vi "PSK_Mod_Receive_queue_simplified.vi"() -> ()   [LabVIEW 2014]
uses:
  <vilib>/addons/Modulation/Digital/General/MT Generate Bits (Galois, PN Order).vi
  <vilib>/Analysis/2dsp.llb/1D Auto Correlation (DBL).vi
  <vilib>/addons/Modulation/Digital/Support/Common/Validators/mod_Generate Bits Validate.vi
  <vilib>/addons/Modulation/Analog/support/mod_Set Error Source.vi
  <vilib>/addons/Modulation/Digital/General/MT Generate PSK System Parameters(M).vi
  <vilib>/addons/Modulation/Digital/Support/Common/Validators/mod_Generate Filter Coefficients Validate.vi
  <vilib>/addons/Modulation/Digital/General/subVIs/mod_Generate Filter Coefficients.vi
  <vilib>/addons/Modulation/Digital/General/subVIs/mod_Generate Bits PN Sequence.vi
  <vilib>/addons/Modulation/Digital/General/MT Generate PSK Synchronization Parameters (bit array).vi
  <instrlib>/niUSRP/niUSRP Fetch Rx Data (CDB Cluster).vi
  <vilib>/addons/Modulation/Digital/General/MT Align to Ideal Symbols (Generic).vi
  <vilib>/addons/Modulation/Digital/General/MT Map PSK Symbols to Bits.vi
  <vilib>/Analysis/2dsp.llb/1D Cross Correlation (DBL).vi
  <vilib>/Utility/file.llb/Write To Spreadsheet File (I64).vi
  <vilib>/addons/Modulation/niDMT.lvlib
  <vilib>/Analysis/NI_AALPro.lvlib
panel:
  in  "stop 2":bool
  out "output bit stream":i8[](array[numeric])
  out "max index(es)":i32
  out "Bits received":i32
  out "Max Rxx Sync Sequence":dbl
  out "Numeric":i32
  in  "stop":bool
  out "USRP loop time":dbl
  in  "Header bits":i32=16
  out "Aquisition time":dbl
  in  "Message bits":i32=128
  in  "Sync bits":i32=30
  out "sync correct?":bool
  out "error out":errorcluster={"status"=FALSE, "code"=1074118647, "source"="niUSRP Fetch Rx Data (CDB Cluster).vi<ERR>Overflow: an internal receive buffer has filled before the data could be returned.  Consider reducing the IQ rate, increasing the Fetch rate, or increasing the number of samples per Fetch."}
  in  "USRP IP Address":refnum<k15>="192.168.10.1"
  out "Actual Rx Parameters":T1={"Rx IQ Sampling\nRate [s/sec]"=200000.0, "Rx\nFrequency [Hz]"=915000000.0, "Rx Gain [dB]"=20.0, "Rx Antenna"="RX1"} {"Rx Gain [dB]" format="%#.6p"; "Rx\nFrequency [Hz]" format="%#.6p"; "Rx IQ Sampling\nRate [s/sec]" format="%#.6p"}
  in  "Rx Parameters":T1={"Rx IQ Sampling\nRate [s/sec]"=400000.0, "Rx\nFrequency [Hz]"=5795000000.0, "Rx Gain [dB]"=0.0, "Rx Antenna"="RX1"} {"Rx Gain [dB]" format="%#.6p"; "Rx\nFrequency [Hz]" format="%#.6p"; "Rx IQ Sampling\nRate [s/sec]" format="%#.6p"}
  in  "Packets per burst":i32=20
  in  "filter parameters":T2={"Alpha"=0.5, "Filter Length"=6, "TX Filter"=enum."Root Raised Cos"} {"Alpha" format="%.2f"}
  in  "QPSK System Parameters":T3={"Samples per Symbol"=8, "symbol map"=[], "Differential PSK"=enum."disable", "PSK type"=0} {"PSK type" items=["normal", "shifted", "offset"]; "symbol map" format="%.3f"}
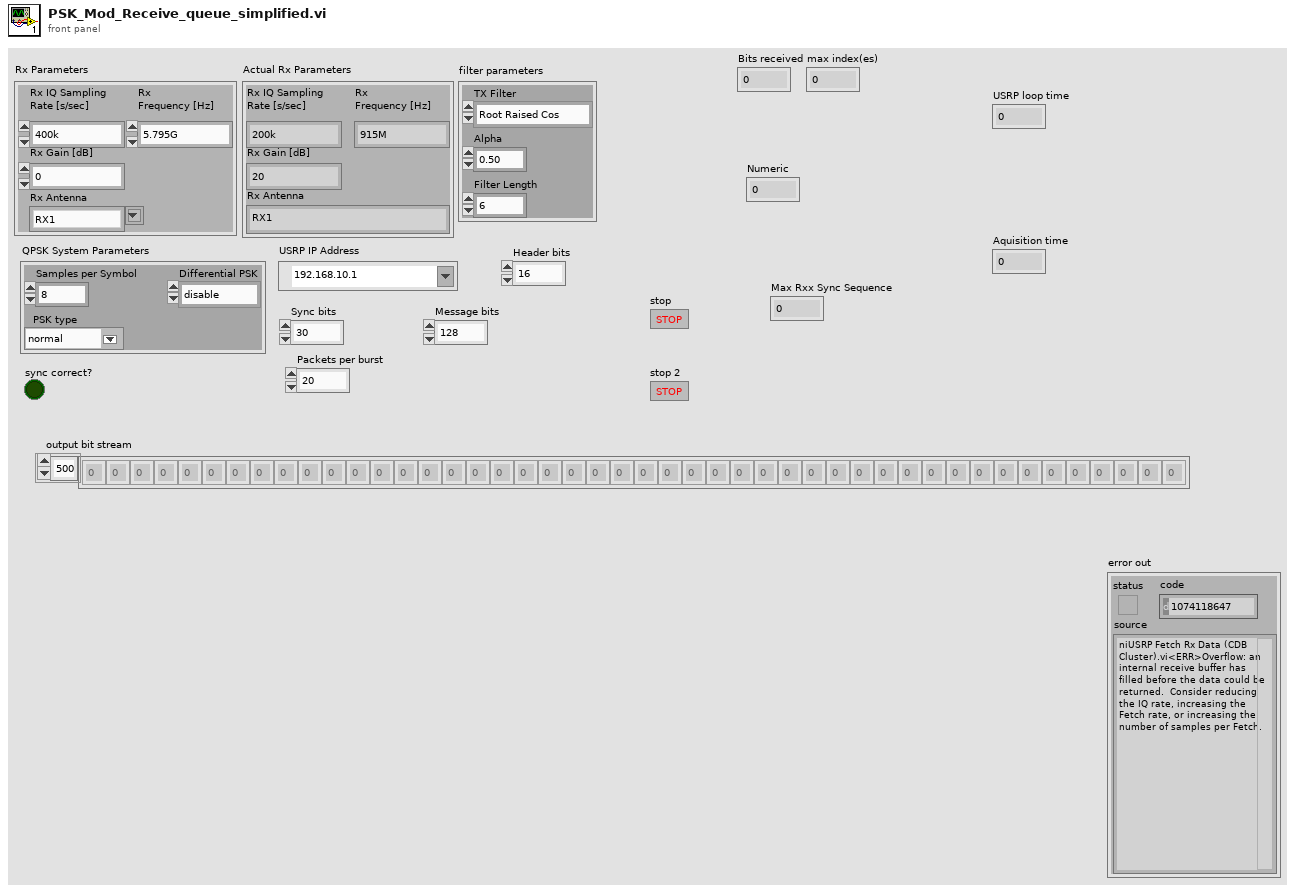
[diagram p1: front panel]
types:
  T1 = cluster{"Rx IQ Sampling\nRate [s/sec]":dbl, "Rx\nFrequency [Hz]":dbl, "Rx Gain [dB]":dbl, "Rx Antenna":string}
  T2 = cluster{"Alpha":dbl, "Filter Length":i32, "TX Filter":enum16{"none", "Raised Cosine", "Root Raised Cos", "Gaussian"}}
  T3 = cluster{"Samples per Symbol":i32, "symbol map":cdb[], "Differential PSK":enum16{"disable", "enable"}, "PSK type":u16}
  T4 = enum16{"FSK", "PSK", "QAM", "MSK", "PAM", "ASK", "CPM"}
  T5 = enum16{"none", "Raised Cosine", "Root Raised Cos", "Gaussian"}
  T6 = cluster{"samples per symbol (16)":i32, "symbol map":cdb[], "differential PSK":enum16{"disable", "enable"}, "PSK type":u16}
  T7 = cluster{"expected sync location (symbols)":i32, "sync sequence":cdb[], "sync location uncertainty (symbols)":i32, "sync indent (symbols)":i32}
  T8 = typedef "niAMT.lvlib/Complex Data Waveform.ctl" = cluster{"t0":dbl, "dt":dbl, "Y":cdb[]}
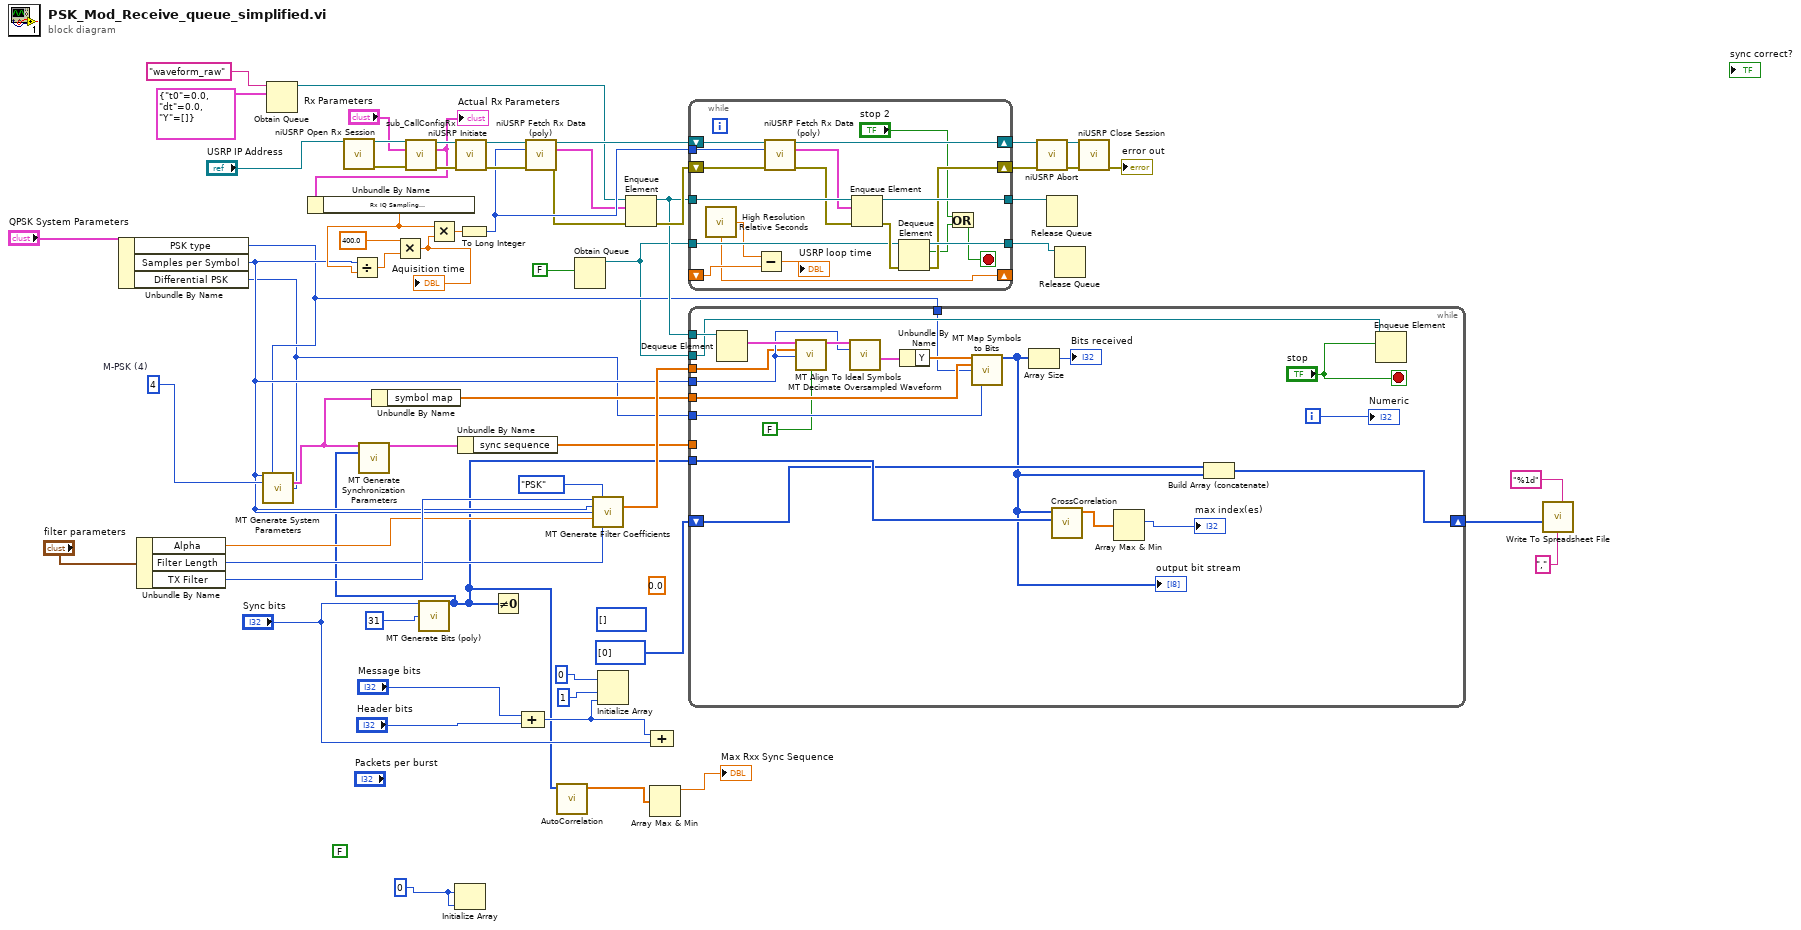
[diagram p0: block diagram]
diagram:
  (unwired) i8[] [] ("output bit stream")
  w25 = 0
  (unwired) FALSE
  (unwired) 0.0
  w19 = 4  # M-PSK (4)
  n1 = Unbundle By Name("QPSK System Parameters") -> ("PSK type"=w13:u16, "Samples per Symbol"=w16:i32, "Differential PSK"=w8:enum16{"disable", "enable"})
  n2 = Unbundle By Name("filter parameters") -> ("Alpha"=w59:dbl, "Filter Length"=w60:i32, "TX Filter"=w61:T5)
  n3 = call-poly <vilib>:"MT Generate System Parameters.vi"("samples per symbol (16)"=w16, "PSK type"=w13, "M-PSK (4)"=w19, "differential PSK"=w8) -> ("PSK system parameters"=w15:T6)  [unwired: 9 in, 2 out]
  n4 = Obtain Queue(name (unnamed)="waveform_raw", element data type=cluster{"t0":dbl, "dt":dbl, "Y":cdb[]} {"t0"=0.0, "dt"=0.0, "Y"=[]} ("data")) -> (queue out=w24:refnum<queue>)  [unwired: 3 in, 2 out]
  n5 = call <instrlib>:"niUSRP Open Rx Session.vi"("device names"="USRP IP Address") -> ("session handle out"=w55:refnum<k15>, "error out"=w56:errorcluster)  [unwired: 13 in]
  n6 = Unbundle By Name(w15) -> ("symbol map"=w14:cdb[])
  n7 = call "sub_CallConfigRx.vi"("session handle"=w55, "Rx Parameters"="Rx Parameters", "error in"=w56) -> ("session handle out"=w53:refnum<k15>, "Actual Rx Parameters"=w50:T1, "error out"=w52:errorcluster)  [unwired: 10 in]
  "Actual Rx Parameters" <- w50
  n8 = Unbundle By Name(w50) -> ("Rx IQ Sampling\nRate [s/sec]"=w20:dbl)
  n9 = Divide(x=w16, y=w20) -> (x/y=w39:dbl)
  n10 = Multiply(x=400.0, y=w39) -> (x*y=w26:dbl)
  "Aquisition time" <- w26
  n11 = call-poly <vilib>:"MT Generate Bits (poly).vi"("total bits (128)"="Sync bits", "PN sequence order (9)"=31) -> ("output bit stream"=w7:i8[])  [unwired: 11 in, 2 out]
  n12 = call-poly <vilib>:"MT Generate Synchronization Parameters.vi"("PSK system parameters"=w15, "sync bits"=w7) -> ("PSK synchronization parameters"=w11:T7)  [unwired: 12 in, 1 out]
  n13 = Multiply(x=w20, y=w26) -> (x*y=w57:dbl)
  n14 = Initialize Array(w25, w25) -> ()  [unwired: 1 out]
  n15 = call <instrlib>:"niUSRP Initiate.vi"("session handle"=w53, "error in (no error)"=w52) -> ("session handle out"=w49:refnum<k15>, "error out"=w48:errorcluster)  [unwired: 12 in]
  n16 = Unbundle By Name(w11) -> ("sync sequence"=w10:cdb[])
  n17 = To Long Integer(number=w57) -> (32bit integer=w41:i32)
  n18 = Not Equal To 0?(x=w7) -> ()  [unwired: 1 out]
  n19 = Compound Arithmetic op=ADD("Message bits", "Header bits") -> (w28:i32)
  n20 = call-poly <instrlib>:"niUSRP Fetch Rx Data (poly).vi"("session handle"=w49, "number of samples"=w41, "error in (no error)"=w48) -> ("session handle out"=w44:refnum<k15>, "data"=w33:cluster{"t0":dbl, "dt":dbl, "Y":cdb[]}, "error out"=w32:errorcluster)  [unwired: 9 in, 1 out]
  n21 = call-poly <vilib>:"AutoCorrelation.vi"("X"=w7) -> ("Rxx"=w6:dbl[])  [unwired: 9 in, 1 out]
  n22 = Obtain Queue(element data type=FALSE) -> (queue out=w12:refnum<queue>)  [unwired: 4 in, 2 out]
  n23 = call <vilib>:"MT Generate Filter Coefficients.vi"("pulse shaping filter (none)"=w61, "modulation type"=T4."PSK", "pulse shaping samples per symbol (16)"=w16, "matched samples per symbol (16)"=w16, "filter parameter"=w59, "filter length (symbols)"=w60) -> ("matched filter coefficients"=w17:dbl[])  [unwired: 7 in, 2 out]
  n24 = Initialize Array(i8 0 ("element"), 1 ("dimension size"), w28) -> ()  [unwired: 1 out]
  n25 = Enqueue Element(queue=w24, element=w33, error in (no error)=w32) -> (queue out=w18:refnum<queue>, error out=w34:errorcluster)  [unwired: 1 in, 1 out]
  n26 = Array Max & Min(array=w6) -> (max value=→"Max Rxx Sync Sequence":dbl)  [unwired: 3 out]
  n27 = Compound Arithmetic op=ADD(w28, "Sync bits") -> ()  [unwired: 1 out]
  n28 = while {
    tunnel: w41 -> [w77]
    shift-right: [w79] -> w43
    shift-left: w44 -> [w80]
    shift-right: [w71] -> w42
    shift-left: w34 -> [w78]
    tunnel: w18 -> [w76]
    tunnel: [w73] -> w30
    tunnel: [w72] -> w9
    tunnel: w12 -> [w69]
    shift-right: [w67] -> _
    shift-left: _ -> [w68]
    stop <- w64 stop-if-true
    n29 = call <vilib>:"High Resolution Relative Seconds.vi"() -> ("relative seconds"=w67:dbl)
    n30 = Subtract(x=w67, y=w68) -> (x-y=→"USRP loop time":dbl)
    n31 = call-poly <instrlib>:"niUSRP Fetch Rx Data (poly).vi"("session handle"=w80, "number of samples"=w77, "error in (no error)"=w78) -> ("session handle out"=w79:refnum<k15>, "data"=w75:cluster{"t0":dbl, "dt":dbl, "Y":cdb[]}, "error out"=w74:errorcluster)  [unwired: 9 in, 1 out]
    n32 = Enqueue Element(queue=w76, element=w75, error in (no error)=w74) -> (queue out=w73:refnum<queue>, error out=w70:errorcluster)  [unwired: 1 in, 1 out]
    n33 = Dequeue Element(queue=w69, error in (no error)=w70) -> (queue out=w72:refnum<queue>, element=w65:bool, error out=w71:errorcluster)  [unwired: 1 in, 1 out]
    n34 = Or(x="stop 2", y=w65) -> (x .or. y?=w64:bool)
  }
  n35 = while {
    tunnel: w18 -> [w101]
    tunnel: w17 -> [w88]
    tunnel: w16 -> [w94]
    tunnel: w14 -> [w92]
    tunnel: w13 -> [w91]
    tunnel: w12 -> [w98]
    tunnel: w10 -> [_]
    tunnel: w8 -> [w90]
    tunnel: w7 -> [w89]
    shift-right: [w82] -> w1
    shift-left: i8[] [0] ("output bit stream 2") -> [w84]
    i -> [w97]
    stop <- "stop" stop-if-true
    n36 = Dequeue Element(queue=w101) -> (element=w96:cluster{"t0":dbl, "dt":dbl, "Y":cdb[]})  [unwired: 2 in, 3 out]
    n37 = call-poly <vilib>:"MT Align To Ideal Symbols.vi"("input complex waveform"=w96, "matched filter coefficients"=w88, "samples per symbol (16)"=w94, "reset? (T)"=FALSE) -> ("output complex waveform"=w95:T8)  [unwired: 9 in, 2 out]
    n38 = call <vilib>:"MT Decimate Oversampled Waveform.vi"("input complex waveform"=w95, "decimation factor"=w94) -> ("output complex waveform"=w100:T8)  [unwired: 12 in, 1 out]
    n39 = Unbundle By Name(w100) -> ("Y"=w93:cdb[])
    n40 = call-poly <vilib>:"MT Map Symbols to Bits.vi"("symbols"=w93, "symbol map"=w92, "PSK type"=w91, "differential PSK"=w90) -> ("output bit stream"=w83:i8[])  [unwired: 10 in, 1 out]
    "output bit stream" <- w83
    n41 = Array Size(array=w83) -> (size(s)=→"Bits received":i32)
    n42 = call-poly <vilib>:"CrossCorrelation.vi"("Y"=w89, "X"=w83) -> ("Rxy"=w86:dbl[])  [unwired: 8 in, 1 out]
    n43 = Array Max & Min(array=w86) -> (max index (indices)=→"max index(es)":i32)  [unwired: 3 out]
    n44 = Build Array (concatenate)(w84, w83) -> (w82:i8[])
    n45 = Enqueue Element(queue=w98, element="stop") -> ()  [unwired: 2 in, 3 out]
    "Numeric" <- w97
  }
  n46 = call <instrlib>:"niUSRP Abort.vi"("session handle"=w43, "error in (no error)"=w42) -> ("session handle out"=w46:refnum<k15>, "error out"=w47:errorcluster)  [unwired: 12 in]
  n47 = Release Queue(queue=w30) -> ()  [unwired: 2 in, 3 out]
  n48 = Release Queue(queue=w9) -> ()  [unwired: 2 in, 3 out]
  n49 = call <instrlib>:"niUSRP Close Session.vi"("session handle"=w46, "error in (no error)"=w47) -> ("error out"=→"error out":errorcluster)  [unwired: 13 in]
  n50 = call-poly <vilib>:"Write To Spreadsheet File.vi"("delimiter (\\t)"="," ("delimiter (\\t)"), "format (%d)"="%1d" ("format (%.3f)"), "1D data"=w1) -> ()  [unwired: 5 in, 1 out]
